vi "niRFUtil RFHS Channelizer ChannelizerRef CSG.vi"(0 "Channelizer Ref":refnum<data-value>, 1 "Reset":bool, 2 "Benchmark Task":T1, 5 "Source Channelizer Ref":refnum<data-value>, 7 "Length":i32=-1, 9 "Channnel":i32, 11 "error in (no error)":errorcluster, 13 "CPU Context":string) -> (4 "Channelizer Ref (out)":refnum<data-value>, 6 "Channel Data":csg[](array[numeric]), 8 "Channel Data Len":u32[](array[numeric]), 15 "error out":errorcluster)   [LabVIEW 2015, in "niRFUtil.lvlib"]
uses:
  niRFUtil.lvlib
  Utilities/Benchmark/niRFUtil RFHS Benchmark Task.ctl
  Includes/niRFUtil RFHS Channelizer ChannelizerInfo CSG.ctl
  Includes/niRFUtil RFHS Channelizer FilterRef.ctl
  Includes/niRFUtil RFHS Channelizer ChannelizerBufferingMode.ctl
  Utilities/Data FIFO/niRFUtil RFHS FIFO Reference.ctl
  Utilities/Data FIFO/niRFUtil RFHS FIFO.ctl
  Includes/niRFUtil RFHS Channelizer ChannelizerType.ctl
  Includes/niRFUtil RFHS Channelizer ChannelizerFlags.ctl
  Includes/niRFUtil RFHS Channelizer Ref.ctl
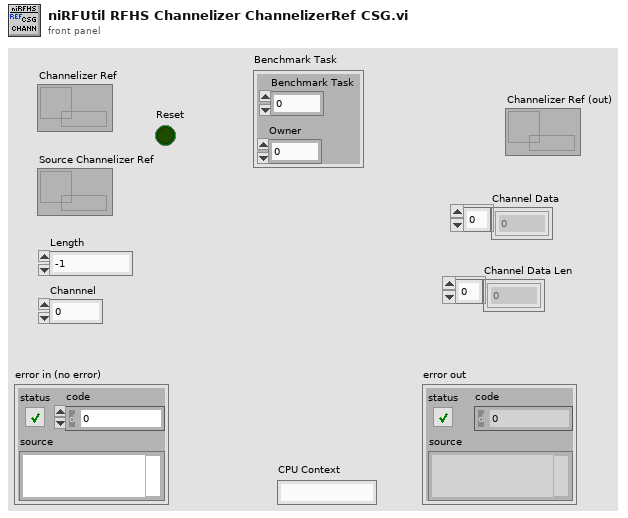
[diagram p1: front panel]
types:
  T1 = typedef "niRFUtil.lvlib/niRFUtil RFHS Benchmark Task.ctl" = cluster{"Benchmark Task":u64, "Owner":u32}
  T2 = typedef "niRFUtil.lvlib/niRFUtil RFHS Channelizer Ref.ctl" = refnum<data-value>
  T3 = typedef "niRFUtil.lvlib/niRFUtil RFHS Channelizer ChannelizerInfo CSG.ctl" = cluster{"Filter LVRef":T4, "Mode":T5, "History":csg[], "Buffer":csg[], "FIFO":T6, "History Len":u32, "Float Cache":csg[], "Double Cache":cdb[], "Type":T8, "Resample Phase":dbl, "fft1Descriptors":u64[], "fft2Descriptors":u64[], "FFT tBuf":csg[], "guardBandLen":i32, "FFT History":csg[], "FFT History Len":u32, "FFTInitDone":u32, "FFT Filter LVRefs":T4[], "FFT fc Offs":u32[], "fft2Sizes":u32[], "BufferW":u32[], "BufferR":u32[], "Buff Off":u32[], "Phase0 (fshift)":dbl[], "Phase (fshift)":dbl[], "fs phase step":dbl[], "Resample Step":dbl, "Flags":T9, "Reset Cnt":i64, "Filter Pass":u32, "Stages":variant[]}
  T4 = typedef "niRFUtil.lvlib/niRFUtil RFHS Channelizer FilterRef.ctl" = cluster{"Ref":u64, "GUID":u64, "Upsample":i32, "Downsample":i32, "Size":i32, "Num Taps":i32}
  T5 = typedef "niRFUtil.lvlib/niRFUtil RFHS Channelizer ChannelizerBufferingMode.ctl" = enum32{"Unbuffered", "Finite", "Continuous"}
  T6 = typedef "niRFUtil.lvlib/niRFUtil RFHS FIFO Reference.ctl" = cluster{"Read Lock":refnum<data-value>, "Info":T7, "Write Lock":refnum<data-value>}
  T7 = typedef "niRFUtil.lvlib/niRFUtil RFHS FIFO.ctl" = cluster{"ID":u64, "Length":u32}
  T8 = typedef "niRFUtil.lvlib/niRFUtil RFHS Channelizer ChannelizerType.ctl" = enum32{"Auto", "Frequency Shift Only", "Resampler Only"}
  T9 = typedef "niRFUtil.lvlib/niRFUtil RFHS Channelizer ChannelizerFlags.ctl" = u32
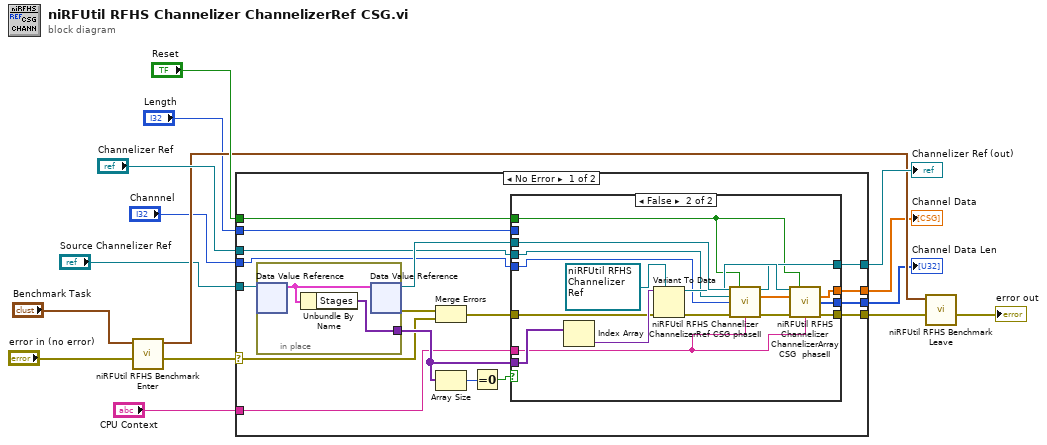
[diagram p0: block diagram]
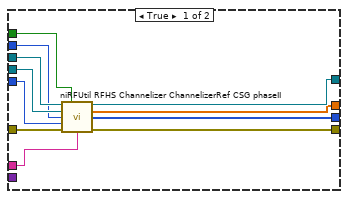
[diagram p2: hidden frame]
diagram:
  n1 = call "niRFUtil RFHS Benchmark Enter.vi"("error in (no error)"="error in (no error)", "Benchmark Task (Parent)"="Benchmark Task") -> ("error out"=w12:errorcluster, "Benchmark Task (Self)"=w6:T1)  [unwired: 8 in]
  n2 = case shown="No Error" w12 {
    selector: w12 -> [w17 w64]
    tunnel: "Reset" -> [w27 _]
    tunnel: [w18 w64] -> w13
    tunnel: "CPU Context" -> [w25 _]
    tunnel: "Channelizer Ref" -> [w24 w63]
    tunnel: [w22 w63] -> w7
    tunnel: "Source Channelizer Ref" -> [w28 _]
    tunnel: "Length" -> [w23 _]
    tunnel: "Channnel" -> [w26 _]
    tunnel: [w21 _] -> w2
    tunnel: [w20 _] -> w1
    frame No Error {
      n3 = in-place {
        in-place-border: [w61] -> w29
        n4 = in-place-dvr #1(w28) -> (w62:T3)  [unwired: 1 out]
        n5 = Unbundle By Name(w62) -> ("Stages"=w61:variant[])
        n6 = in-place-dvr #1(w62) -> (w32:refnum<data-value>, w19:errorcluster)
      }
      n7 = Merge Errors(w19, w17) -> (w16:errorcluster)
      n8 = Array Size(array=w29) -> (size(s)=w31:i32)
      n9 = Equal To 0?(x=w31) -> (x = 0?=w30:bool)
      n10 = case shown="False" w30 {
        tunnel: w16 -> [w43 w52]
        tunnel: [w42 w50] -> w22
        tunnel: [w41 w57] -> w20
        tunnel: w25 -> [w40 w48]
        tunnel: w27 -> [w39 w49]
        tunnel: [w38 w58] -> w21
        tunnel: w32 -> [w37 w60]
        tunnel: w29 -> [_ w56]
        tunnel: w26 -> [w36 w46]
        tunnel: w24 -> [w35 w47]
        tunnel: w23 -> [w34 _]
        tunnel: [w33 w45] -> w18
        frame True {
          n11 = call "niRFUtil RFHS Channelizer ChannelizerRef CSG phaseII.vi"("Channelizer Ref"=w37, "Reset"=w39, "Source Channelizer Ref"=w35, "Length"=w34, "Channnel"=w36, "error in (no error)"=w43, "CPU Context"=w40) -> ("Channelizer Ref (out)"=w42:refnum<data-value>, "Channel Data"=w41:csg[], "Channel Data Len"=w38:u32[], "error out"=w33:errorcluster)  [unwired: 5 in]
        }
        frame False {
          n12 = Index Array(array=w56) -> (element=w55:variant)  [unwired: 1 in]
          n13 = Variant To Data(error in=w52, type=T2 refnum ("Channelizer Ref"), Variant=w55) -> (data=w53:T2, error out=w51:errorcluster)
          n14 = call "niRFUtil RFHS Channelizer ChannelizerRef CSG phaseII.vi"("Channelizer Ref"=w60, "Reset"=w49, "Source Channelizer Ref"=w47, "Length"=w46, "error in (no error)"=w51, "CPU Context"=w48) -> ("Channelizer Ref (out)"=w50:refnum<data-value>, "Channel Data"=w44:csg[], "error out"=w59:errorcluster)  [unwired: 6 in, 1 out]
          n15 = call "niRFUtil RFHS Channelizer ChannelizerArray CSG  phaseII.vi"("Channelizer Ref"=w53, "Reset"=w49, "Data"=w44, "error in (no error)"=w59, "CPU Context"=w48) -> ("Channel Data"=w57:csg[], "Channel Data Len"=w58:u32[], "error out"=w45:errorcluster)  [unwired: 7 in, 1 out]
        }
      }
    }
    frame Error {
    }
  }
  "Channel Data" <- w1
  "Channelizer Ref (out)" <- w7
  "Channel Data Len" <- w2
  n16 = call "niRFUtil RFHS Benchmark Leave.vi"("error in (no error)"=w13, "Benchmark Task Self"=w6) -> ("error out"=→"error out":errorcluster)  [unwired: 8 in, 1 out]
